vi "Acquire Digital Data.vi"   [LabVIEW 2020]
uses:
  Type Definitions/Enum - Data.ctl
  Type Definitions/Payload Class.ctl
  Type Definitions/Digital Input Data.ctl
  <vilib>/Platform/TimedLoop/XDataNode/wakeup.ctl
  <vilib>/Platform/TimedLoop/XDataNode/XDNodeRunTimeDep.lvlib
  <vilib>/Platform/TimedLoop/XDataNode/nitl_modes.ctl
  <vilib>/Platform/TimedLoop/XDataNode/timing_clust.ctl
  <vilib>/platform/TimedLoop/XDataNode/XDataNode.xnode
  <vilib>/rvi/interface/nirviMethod/nirviMethod.xnode
  <vilib>/FPGAPlugInAG/Dynamic/niLvFpga_ReadFifo_Dynamic.vi
  <vilib>/rvi/errors/niLvFpgaMergeErrorWithErrorCode.vi
  <vilib>/rvi/interface/nirviReadWriteControl/nirviReadWriteControl.xnode
  <vilib>/Utility/error.llb/Error Cluster From Error Code.vi
  <vilib>/rvi/interface/Simulation/niFpgaSimulationCallBeginRW.vi
  <vilib>/rvi/errors/niLvFpgaAdjustHostInterfaceError.vi
  NiFpgaLv.dll
  <vilib>/FPGAPlugInAG/Dynamic/niLvFpga_StartFifo_Dynamic.vi
types:
  T1 = typedef "System Resources.ctl" = cluster{"System Session":refnum<k21>, "System Resource":refnum<k20>, "FPGA VI Reference":refnum<k20>}
  T2 = typedef "XDNodeRunTimeDep.lvlib/timing_clust.ctl" = cluster{"Expected End [f-1]":u64, "Actual End [f-1]":u64, "Finished Late? [f-1]":bool, "Expected End [i-1]":u64, "Actual End [i-1]":u64, "Finished Late? [i-1]":bool, "Expected Start [i]":u64, "Actual Start [i]":u64, "Expected Start [f]":u64, "Actual Start [f]":u64, "Source Name":string, "Structure Name":string, "Period":i64, "Deadline":i64, "Offset":i64, "Start":i64, "Priority":i32, "Timeout":i32, "Mode":T3, "Wakeup Reason":T4, "Error":errorcluster, "Source Type":string, "Secondary Source Type":string, "Global End Time":u64, "Global Start Time":u64, "Frame Duration":u64, "Iteration Duration":u64, "Assigned CPU":i32, "I/O Scan Engine Mode":u32}
  T3 = typedef "XDNodeRunTimeDep.lvlib/nitl_modes.ctl" = enum32{"No Change", "Process missed periods, maintain original phase", "Discard missed periods, maintain original phase", "Process missed periods, ignore original phase", "Discard missed periods, ignore original phase"}
  T4 = typedef "XDNodeRunTimeDep.lvlib/wakeup.ctl" = enum32{"Normal", "Aborted", "Asynchronous wakeup", "Timing source error", "Timed loop error", "Timeout"}
  T5 = typedef "Digital Input Data.ctl" = cluster{"Digital Data":u32[][]}
  T6 = typedef "Payload Class.ctl" = enum16{"System State", "Parameters", "Metadata", "Software Monitor", "Data", "Commands"}
  T7 = typedef "Enum - Data.ctl" = enum16{"Analog Input Data", "Notification Data", "Analog Output Data", "Digital Output Data", "Command Ack", "Digital Input Data", "GPS Solution Data"}
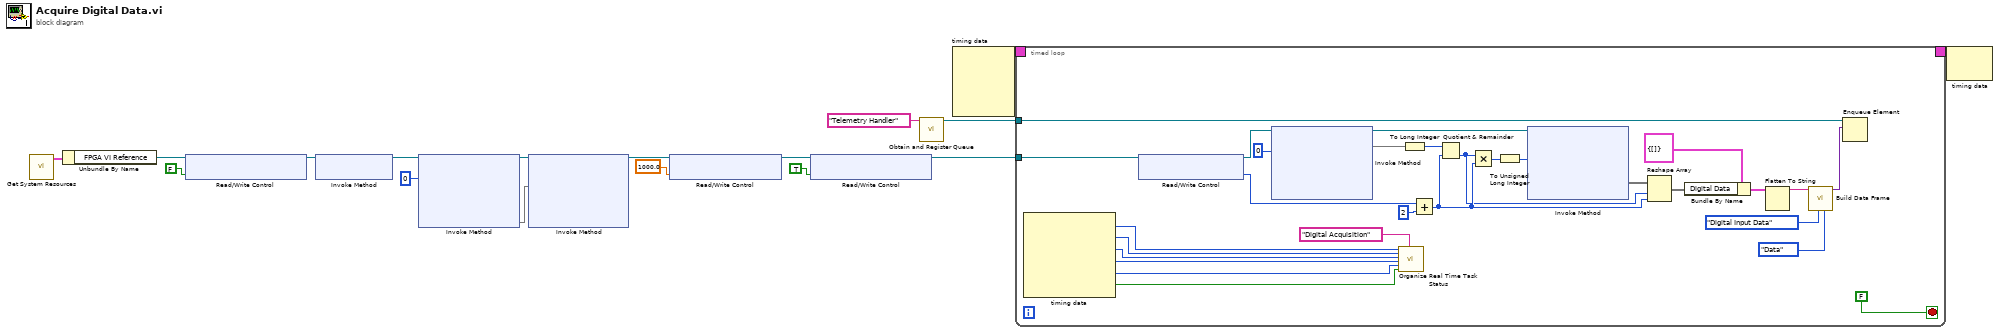
[diagram p0: block diagram]
diagram:
  n1 = call "Get System Resources.vi"() -> ("System Resources"=w1:T1)  [unwired: 10 in, 1 out]
  n2 = Unbundle By Name(w1) -> ("FPGA VI Reference"=w3:refnum<k20>)
  n3 = xnode "Read/Write Control"("FPGA VI Reference In"=w3, "Enable Digital Acquisition"=FALSE) -> ("FPGA VI Reference Out"=w4:refnum<k20>)  [unwired: 1 in, 1 out]
  n4 = xnode "Invoke Method"("FPGA VI Reference In"=w4) -> ("FPGA VI Reference Out"=w5:refnum<k20>)  [unwired: 1 in, 1 out]
  n5 = xnode "Invoke Method"("FPGA VI Reference In"=w5, "Number of Elements"=u32 0) -> ("FPGA VI Reference Out"=w7:refnum<k20>, "Elements Remaining"=w6)  [unwired: 2 in, 2 out]
  n6 = xnode "Invoke Method"("FPGA VI Reference In"=w7, "Number of Elements"=w6) -> ("FPGA VI Reference Out"=w8:refnum<k20>)  [unwired: 2 in, 3 out]
  n7 = xnode "Read/Write Control"("FPGA VI Reference In"=w8, "Digital Acquisition Rate"=sgl 1000.0 ("Acquisition Rate (10,000 Hz)")) -> ("FPGA VI Reference Out"=w9:refnum<k20>)  [unwired: 1 in, 1 out]
  n8 = xnode "Read/Write Control"("FPGA VI Reference In"=w9, "Enable Digital Acquisition"=TRUE) -> ("FPGA VI Reference Out"=w10:refnum<k20>)  [unwired: 1 in, 1 out]
  n9 = call "Obtain and Register Queue.vi"("name (unnamed)"="Telemetry Handler") -> ("Queue Out"=w2:refnum<queue>)  [unwired: 7 in, 3 out]
  n10 = node-c288() -> (w17:T2)  [unwired: 4 in]
  n11 = timed-loop {
    timing: w17 -> [_]
    timing-out: [_] -> w16
    tunnel: w2 -> [w24]
    tunnel: w10 -> [w37]
    stop <- FALSE stop-if-true
    n12 = node-c288() -> (w44:i32, w43:i32, w42:i64, w41:i64, w40:i64, w39:bool)  [unwired: 1 in]
    n13 = xnode "Read/Write Control"("FPGA VI Reference In"=w37) -> ("FPGA VI Reference Out"=w29:refnum<k20>, "Digital Module Count"=w30:i32)  [unwired: 1 in, 1 out]
    n14 = xnode "Invoke Method"("FPGA VI Reference In"=w29, "Number of Elements"=u32 0) -> ("FPGA VI Reference Out"=w33:refnum<k20>, "Elements Remaining"=w35)  [unwired: 2 in, 2 out]
    n15 = call "Organize Real Time Task Status.vi"("Priority"=w44, "Processor"=w43, "Offset"=w42, "Iteration Duration"=w41, "Period"=w40, "Finished Late? [i-1]"=w39, "Task Name"="Digital Acquisition") -> ()  [unwired: 12 in, 1 out]
    n16 = To Long Integer(number=w35) -> (32bit integer=w34:i32)
    n17 = Add(x=w30, y=2) -> (x+y=w31:i32)
    n18 = Quotient & Remainder(x=w34, y=w31) -> (floor(x/y)=w28:i32)  [unwired: 1 out]
    n19 = Multiply(x=w28, y=w31) -> (x*y=w19:i32)
    n20 = To Unsigned Long Integer(number=w19) -> (unsigned 32bit integer=w18:u32)
    n21 = xnode "Invoke Method"("FPGA VI Reference In"=w33, "Number of Elements"=w18) -> ("Data"=w32:void[])  [unwired: 2 in, 3 out]
    n22 = Reshape Array(w32, w28, w31) -> (w21:void[][])
    n23 = Bundle By Name(cluster=T5 {"Digital Data"=[]} ("Digital Input Data"), "Digital Data"=w21) -> (w22:T5)
    n24 = Flatten To String(anything=w22) -> (data string=w27:string)  [unwired: 3 in, 2 out]
    n25 = call "Build Data Frame.vi"("Payload Class (Data)"=Payload_Class."Data", "Payload ID (0)"=Enum_-_Data."Digital Input Data" ("Data"), "Payload (Empty String)"=w27) -> ("Frame"=w23:variant)  [unwired: 7 in, 1 out]
    n26 = Enqueue Element(queue=w24, element=w23) -> ()  [unwired: 2 in, 3 out]
  }
  n27 = node-c288(w16) -> ()  [unwired: 1 out]
